vi "Camera Create.vi"(8 "error in (no error)":errorcluster, 10 "Python Session In":refnum<k35>, 11 "Camera in":refnum<class "Camera.lvclass">) -> (0 "error out":errorcluster, 3 "Camera out":refnum<class "Camera.lvclass">)   [LabVIEW 2018, in "Camera Library.lvlib" / "Camera.lvclass"]
uses:
  Camera.lvclass
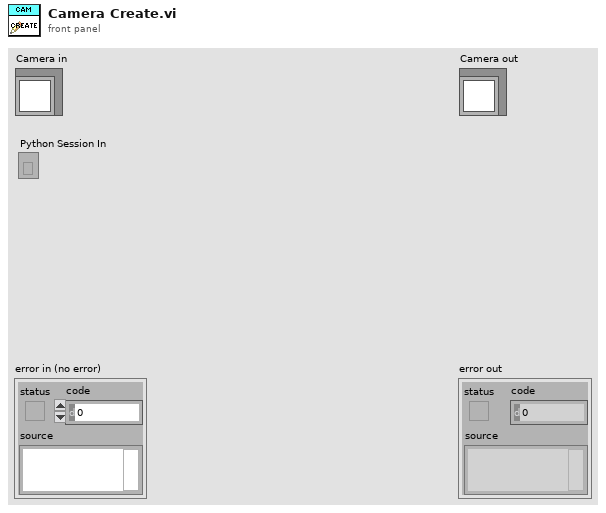
[diagram p1: front panel]
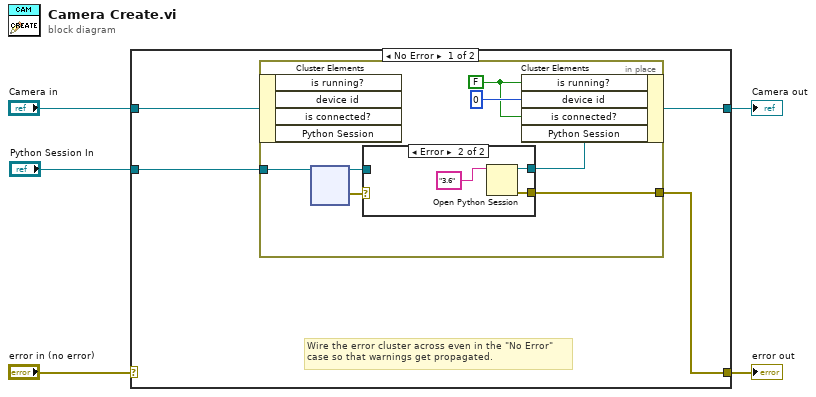
[diagram p0: block diagram]
diagram:
  n1 = case shown="No Error" "error in (no error)" {
    selector: "error in (no error)" -> [_ w23]
    tunnel: [w6 w23] -> w4
    tunnel: [w8 w22] -> w2
    tunnel: "Camera in" -> [w9 w22]
    tunnel: "Python Session In" -> [w7 _]
    frame No Error {
      # "Wire the error cluster across even in the \"No Error\"\ncase so that warnings get propagated."
      n2 = in-place {
        in-place-border: w7 -> [w14]
        in-place-border: [w10] -> w6
        w15 = FALSE ("is running?")
        n3 = in-place-cluster #1(w9) -> ()  [unwired: 4 out]
        n4 = node(w14) -> (w11:refnum<k35>, w13:errorcluster)  [unwired: 5 in, 2 out]
        n5 = case shown="Error" w13 {
          selector: w13 -> [w17 _]
          tunnel: [w18 w21] -> w12
          tunnel: w11 -> [w18 _]
          tunnel: [w17 w19] -> w10
          frame No Error {
          }
          frame Error {
            n6 = Open Python Session(python version="3.6" ("Python version")) -> (session out=w21:refnum<k35>, error out=w19:errorcluster)  [unwired: 2 in]
          }
        }
        n7 = in-place-cluster #1("is running?"=w15, "device id"=u32 0, "is connected?"=w15, "Python Session"=w12) -> (w8:refnum<class "Camera.lvclass">)
      }
    }
    frame Error {
    }
  }
  "error out" <- w4
  "Camera out" <- w2
